vi "GetConfig.vi"(8 "error in (no error)":errorcluster, 11 "Sim in":refnum<class "TestView_Base.lvclass">) -> (0 "error out":errorcluster, 2 "Config XML":string, 3 "Sim out":refnum<class "TestView_Base.lvclass">)   [LabVIEW 2017]
uses:
  TestView_Base.lvclass
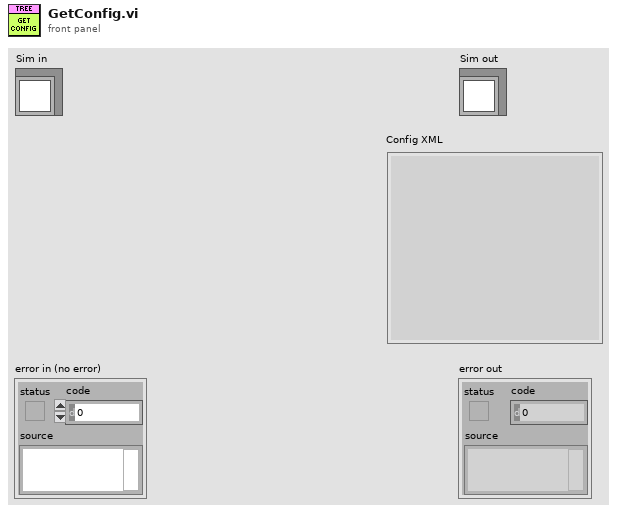
[diagram p1: front panel]
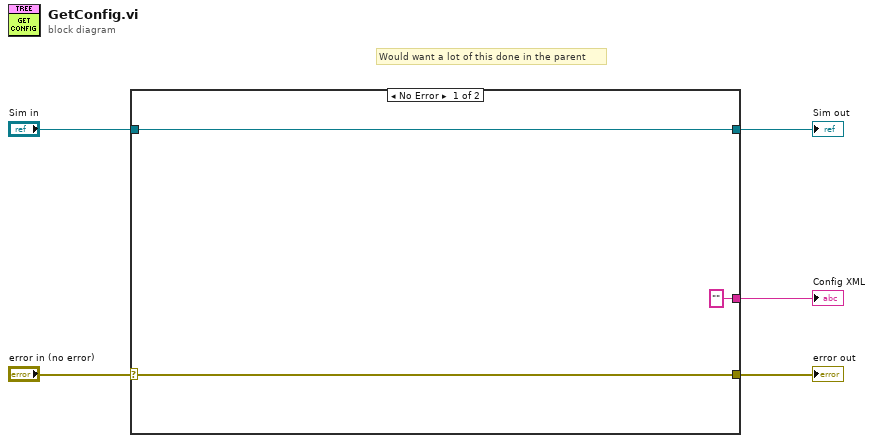
[diagram p0: block diagram]
diagram:
  # "Would want a lot of this done in the parent"
  n1 = case shown="No Error" "error in (no error)" {
    selector: "error in (no error)" -> [w8 w10]
    tunnel: [w8 w10] -> w4
    tunnel: [w6 w9] -> w2
    tunnel: "Sim in" -> [w6 w9]
    tunnel: ["" _] -> w1
    frame No Error {
    }
    frame Error {
    }
  }
  "error out" <- w4
  "Sim out" <- w2
  "Config XML" <- w1
